vi "Set NISync Plugin Timekeeper.vi"(8 "error in (no error)":errorcluster, 11 "RT Data Cluster in":T1={"Timekeeper hdl"="", "clkDisc session"=variant, "Compiled Data"={"SyncMod?"=FALSE, "SyncMod"="", "ConnectionSettings"={"Mode"=enum."Generate sample clock", "pxitrig"=FALSE, "pfi0"=FALSE, "pfi1"=FALSE, "pfi2"=FALSE, "External Pin"=enum."PFI0", "Routes"=[]}, "TimeKeeper"="", "ScanOffset(%)"=0.0, "StartDelay(s)"=0, "Time Ref Settings"={"Time Reference"=enum."GPS", "Priority 1"=0, "Priority 2"=0, "IRIG type"=enum."IRIGB AM", "Terminal"="", "PPSSetTime"=FALSE, "Start Time"=timestamp(0 s since 1904-01-01)}, "FIFO Locations"={"SysTime"=[], "TimeRef"=[], "Status"=[]}}, "OutputsData"=[], "OutputsFIFO"=refnum, "Scan Period"=0, "Timekeeper type"=enum."6683", "SyncMod type"=enum."6683", "SyncMod hdl"=""} {"Compiled Data"."Time Ref Settings"."Priority 2" min=0 max=255; "Compiled Data"."Time Ref Settings"."Priority 1" min=0 max=255}) -> (0 "error out":errorcluster, 3 "RT Data Cluster out":T1={"Timekeeper hdl"="", "clkDisc session"=variant, "Compiled Data"={"SyncMod?"=FALSE, "SyncMod"="", "ConnectionSettings"={"Mode"=enum."Generate sample clock", "pxitrig"=FALSE, "pfi0"=FALSE, "pfi1"=FALSE, "pfi2"=FALSE, "External Pin"=enum."PFI0", "Routes"=[]}, "TimeKeeper"="", "ScanOffset(%)"=0.0, "StartDelay(s)"=0, "Time Ref Settings"={"Time Reference"=enum."GPS", "Priority 1"=0, "Priority 2"=0, "IRIG type"=enum."IRIGB AM", "Terminal"="", "PPSSetTime"=FALSE, "Start Time"=timestamp(0 s since 1904-01-01)}, "FIFO Locations"={"SysTime"=[], "TimeRef"=[], "Status"=[]}}, "OutputsData"=[], "OutputsFIFO"=refnum, "Scan Period"=0, "Timekeeper type"=enum."6683", "SyncMod type"=enum."6683", "SyncMod hdl"=""} {"Compiled Data"."Time Ref Settings"."Priority 2" min=0 max=255; "Compiled Data"."Time Ref Settings"."Priority 1" min=0 max=255})   [LabVIEW 2015, in "Chassis TimeSync Engine.lvlib"]
uses:
  Chassis TimeSync Engine.lvlib
  RT Data Cluster.ctl
  mdevClkDisc.llb/_clkDisc_session.ctl
  Shared/Compiled Data.ctl
  Shared/Connection Settings.ctl
  Shared/Mode.ctl
  Shared/External Pin.ctl
  Shared/Routes.ctl
  Shared/Route.ctl
  Shared/Time Ref Settings.ctl
  Shared/Time Reference.ctl
  Shared/IRIG Type.ctl
  timekeeper type.ctl
  <vilib>/Utility/config.llb/Write Key (String).vi
  <vilib>/Utility/config.llb/Read Key (String).vi
  <vilib>/Utility/config.llb/NI_LVConfig.lvlib
  Shared/Chassis TimeSync Shared.lvlib
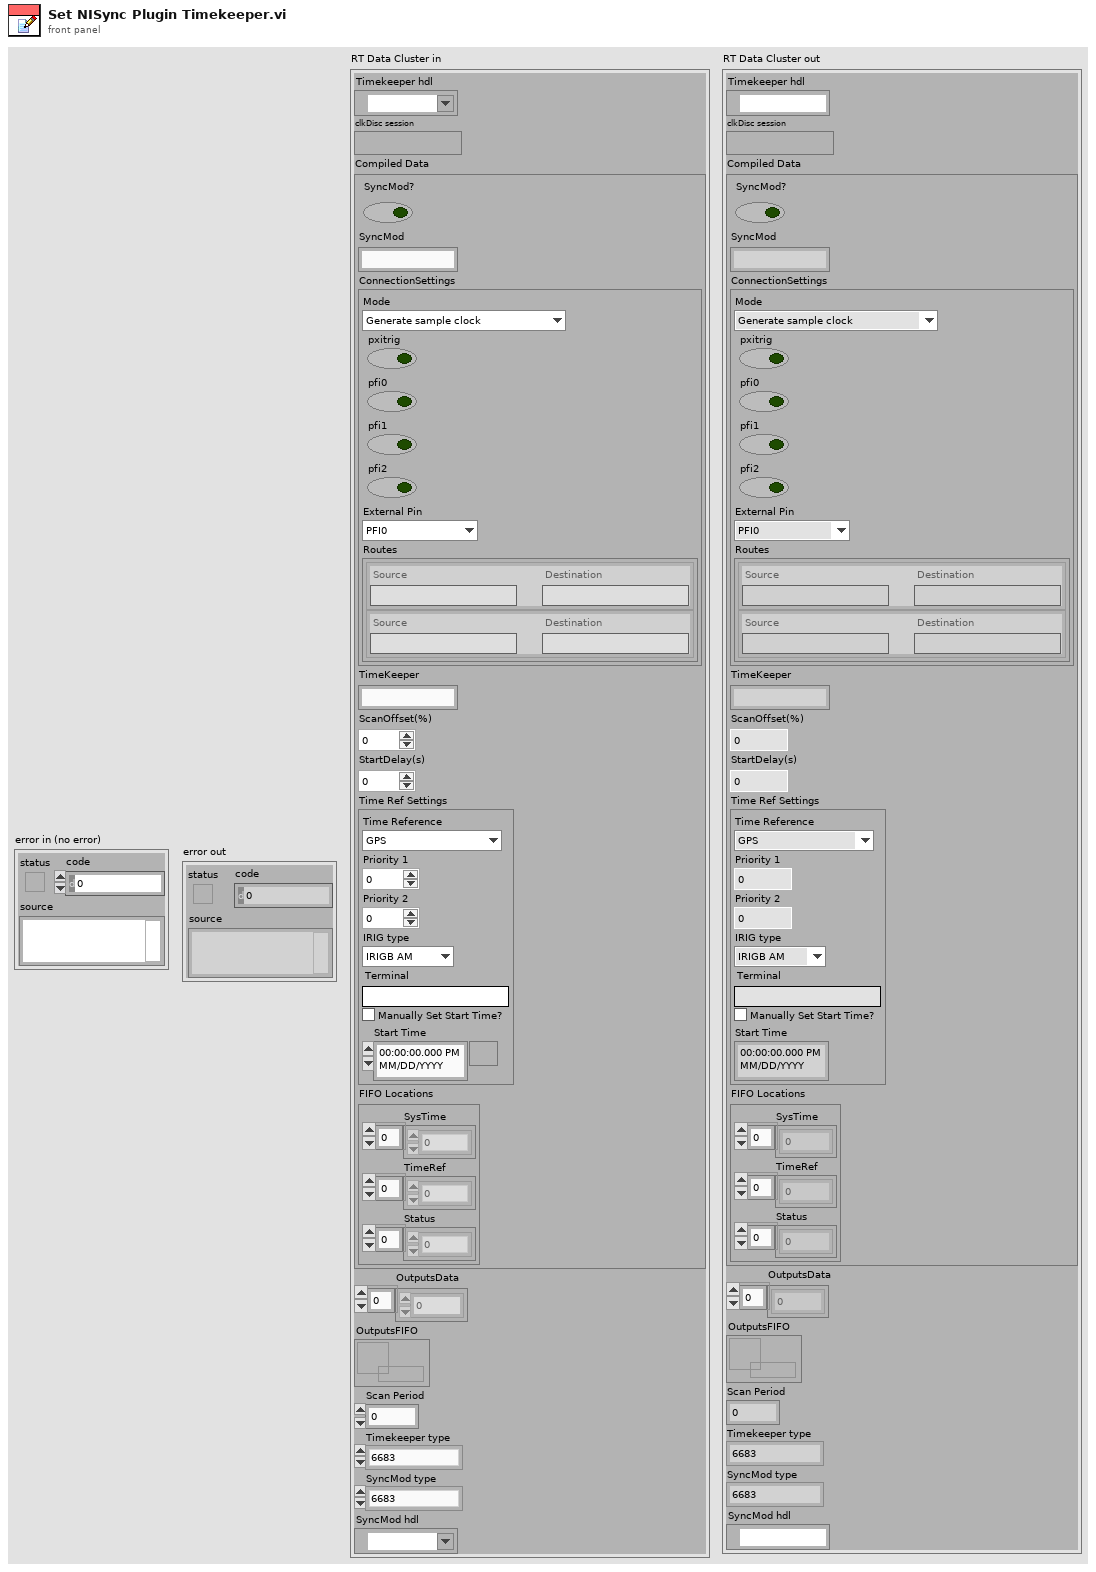
[diagram p1: front panel]
types:
  T1 = typedef "Chassis TimeSync Engine.lvlib/RT Data Cluster.ctl" = cluster{"Timekeeper hdl":refnum<k15>, "clkDisc session":T2, "Compiled Data":T3, "OutputsData":dbl[], "OutputsFIFO":refnum<k33>, "Scan Period":u32, "Timekeeper type":T12, "SyncMod type":T12, "SyncMod hdl":refnum<k15>}
  T2 = typedef "_clkDisc_session.ctl" = variant
  T3 = typedef "Chassis TimeSync Shared.lvlib/Compiled Data.ctl" = cluster{"SyncMod?":bool, "SyncMod":string, "ConnectionSettings":T4, "TimeKeeper":string, "ScanOffset(%)":dbl, "StartDelay(s)":u16, "Time Ref Settings":T9, "FIFO Locations":cluster{"SysTime":i32[], "TimeRef":i32[], "Status":i32[]}}
  T4 = typedef "Chassis TimeSync Shared.lvlib/Connection Settings.ctl" = cluster{"Mode":T5, "pxitrig":bool, "pfi0":bool, "pfi1":bool, "pfi2":bool, "External Pin":T6, "Routes":T7}
  T5 = typedef "Chassis TimeSync Shared.lvlib/Mode.ctl" = enum16{"Generate sample clock", "Route sample clock out of chassis", "Route sample clock into chassis", "Custom routes"}
  T6 = typedef "Chassis TimeSync Shared.lvlib/External Pin.ctl" = enum16{"PFI0", "PFI1", "PFI2"}
  T7 = typedef "Chassis TimeSync Shared.lvlib/Routes.ctl" = T8[]
  T8 = typedef "Chassis TimeSync Shared.lvlib/Route.ctl" = cluster{"Source":string, "Destination":string}
  T9 = typedef "Chassis TimeSync Shared.lvlib/Time Ref Settings.ctl" = cluster{"Time Reference":T10, "Priority 1":i32, "Priority 2":i32, "IRIG type":T11, "Terminal":string, "PPSSetTime":bool, "Start Time":timestamp}
  T10 = typedef "Chassis TimeSync Shared.lvlib/Time Reference.ctl" = enum16{"GPS", "IRIG", "PPS", "1588 Ordinary Clock", "PXI Chassis Clock", "Free Running (Internal)"}
  T11 = typedef "Chassis TimeSync Shared.lvlib/IRIG Type.ctl" = enum16{"IRIGB DC", "IRIGB AM"}
  T12 = typedef "Chassis TimeSync Engine.lvlib/timekeeper type.ctl" = enum16{"6683", "6683H", "6682", "6682H", "non-timekeeper", "timekeeper"}
  T13 = typedef "NI_LVConfig.lvlib/Config Data RefNum.ctl" = refnum<k1>
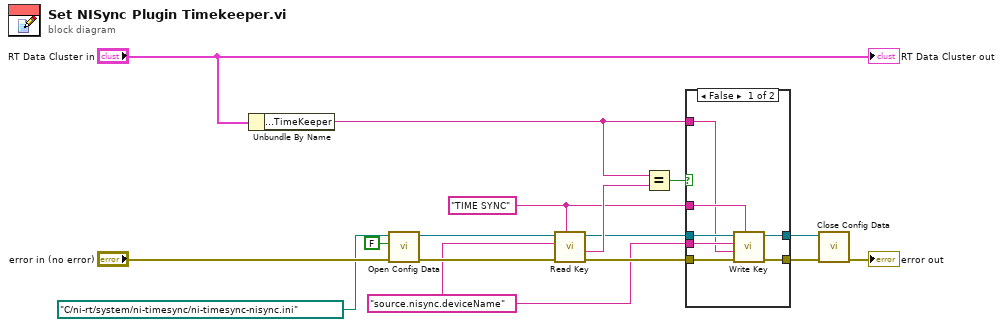
[diagram p0: block diagram]
diagram:
  w5 = "source.nisync.deviceName" ("section")
  w6 = "TIME SYNC" ("section")
  n1 = Unbundle By Name("RT Data Cluster in") -> ("Compiled Data.TimeKeeper"=w4:string)
  n2 = call <vilib>:"Open Config Data.vi"("error in (no error)"="error in (no error)", "create file if necessary (T)"=FALSE, "configuration file path"=path "C:/ni-rt/system/ni-timesync/ni-timesync-nisync.ini") -> ("error out"=w13:errorcluster, "refnum"=w12:T13)  [unwired: 6 in, 1 out]
  n3 = call-poly <vilib>:"Read Key.vi"("section"=w6, "error in (no error)"=w13, "key"=w5, "refnum"=w12) -> ("error out"=w11:errorcluster, "value"=w10:string, "refnum out"=w7:T13)  [unwired: 4 in, 1 out]
  n4 = Equal?(x=w4, y=w10) -> (x = y?=w8:bool)
  n5 = case shown="False" w8 {
    tunnel: w11 -> [w23 w24]
    tunnel: w7 -> [w22 w25]
    tunnel: w6 -> [w21 _]
    tunnel: w5 -> [w20 _]
    tunnel: w4 -> [w19 _]
    tunnel: [w18 w24] -> w3
    tunnel: [w17 w25] -> w2
    frame False {
      n6 = call-poly <vilib>:"Write Key.vi"("section"=w21, "error in (no error)"=w23, "value"=w19, "key"=w20, "refnum"=w22) -> ("error out"=w18:errorcluster, "refnum out"=w17:T13)  [unwired: 4 in, 1 out]
    }
    frame True {
    }
  }
  n7 = call <vilib>:"Close Config Data.vi"("error in (no error)"=w3, "refnum"=w2) -> ("error out"=→"error out":errorcluster)  [unwired: 8 in, 1 out]
  "RT Data Cluster out" <- "RT Data Cluster in"
